vi "Generate Node list.vi"(10 "error in":errorcluster, 11 "Node-Dep Cluster":T1[](array[typedef])) -> (2 "error out":errorcluster, 3 "Node List":string)   [LabVIEW 2018, in "Name and Dependency Processing.lvlib"]
uses:
  Name and Dependency Processing.lvlib
  Name - Dep Cluster.ctl
  DGML Creation/Create Node String.vi
  Path and string processing/Create Array from FQN.vi
  Path and string processing/Determine if name or container.vi
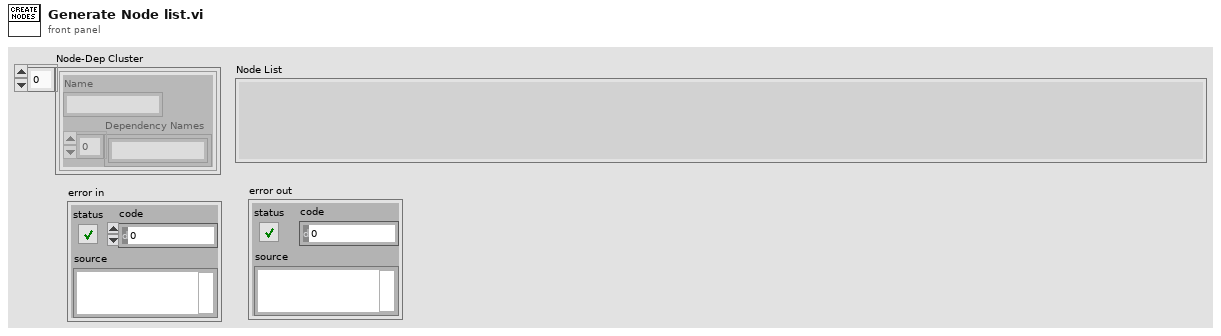
[diagram p1: front panel]
types:
  T1 = typedef "Name and Dependency Processing.lvlib/Name - Dep Cluster.ctl" = cluster{"Name":string, "Dependency Names":string[]}
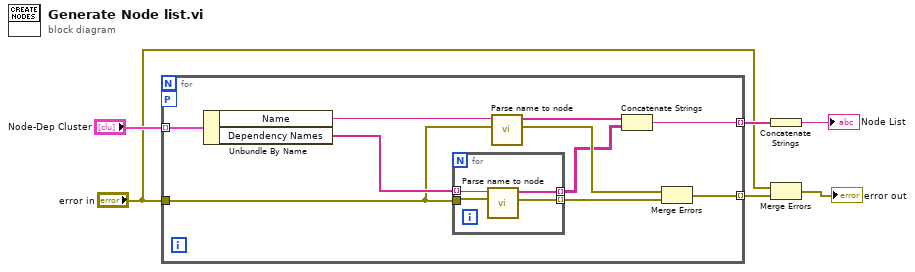
[diagram p0: block diagram]
diagram:
  n1 = for {
    tunnel: "Node-Dep Cluster" -> [w16] mode=indexing
    tunnel: [w12] -> w6 mode=indexing
    workers-P: _ -> [_]
    tunnel: "error in" -> [w11]
    tunnel: [w8] -> w3 mode=indexing
    n2 = Unbundle By Name(w16) -> ("Name"=w15:string, "Dependency Names"=w14:string[])
    n3 = for {
      tunnel: w14 -> [w20] mode=indexing
      tunnel: [w19] -> w7 mode=indexing
      tunnel: w11 -> [w18]
      tunnel: [w17] -> w9 mode=indexing
      n4 = call "Parse name to node.vi"("error in"=w18, "Name"=w20) -> ("error out"=w17:errorcluster, "Array"=w19:string[])  [unwired: 8 in]
    }
    n5 = call "Parse name to node.vi"("error in"=w11, "Name"=w15) -> ("error out"=w10:errorcluster, "Array"=w13:string[])  [unwired: 8 in]
    n6 = Concatenate Strings(w13, w7) -> (w12:string)
    n7 = Merge Errors(w10, w9) -> (w8:errorcluster)
  }
  n8 = Concatenate Strings(w6) -> (→"Node List":string)
  n9 = Merge Errors("error in", w3) -> (→"error out":errorcluster)
